vi "Global_Wait_Asnwer(SubVI).vi"(10 "Wait_answer":bool=TRUE, 11 "R/W":T1) -> (2 "Wait_answer":bool)   [LabVIEW 2015]
uses:
  R_W.ctl
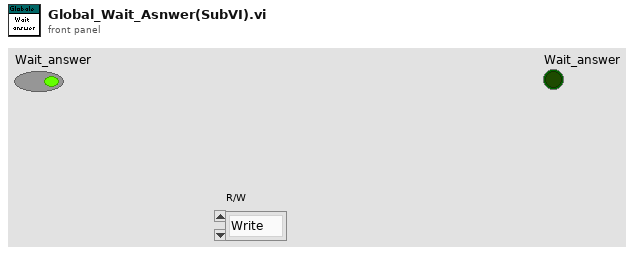
[diagram p1: front panel]
types:
  T1 = typedef "R_W.ctl" = enum16{"Write", "Read", "RAZ"}
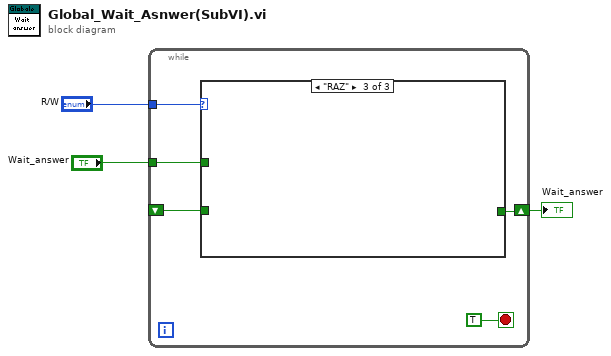
[diagram p0: block diagram]
diagram:
  n1 = while {
    tunnel: "R/W" -> [w8]
    shift-right: [w6] -> w1
    shift-left: _ -> [w5]
    tunnel: "Wait_answer" -> [w4]
    stop <- TRUE stop-if-true
    n2 = case shown="\"RAZ\"" w8 {
      tunnel: [w9 w10 _] -> w6
      tunnel: w5 -> [_ w10 _]
      tunnel: w4 -> [w9 _ _]
      frame "Write", Default {
      }
      frame "Read" {
      }
      frame "RAZ" {
      }
    }
  }
  "Wait_answer" <- w1
